vi "Edit.vi"(8 "error in (no error)":errorcluster, 10 "Edit dialog":T1, 11 "Action in":refnum<class "Substrate.lvclass">) -> (0 "error out":errorcluster, 3 "Action out":refnum<class "Substrate.lvclass">)   [LabVIEW 2013, in "PowderDeposition.lvlib" / "Substrate.lvclass"]
uses:
  Substrate.lvclass
  Move-Absolute/Move-Absolute-settings.ctl
  Substrate.lvclass/Substrate.ctl
  Move-Absolute/Move-Absolute.lvclass
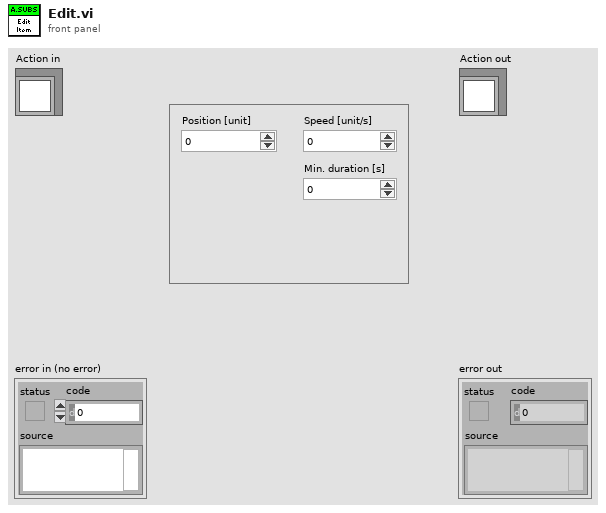
[diagram p1: front panel]
types:
  T1 = typedef "PowderDeposition.lvlib/Move-Absolute.lvclass/Move-Absolute-settings.ctl" = cluster{"Position":dbl, "Speed":dbl, "Min duration":dbl}
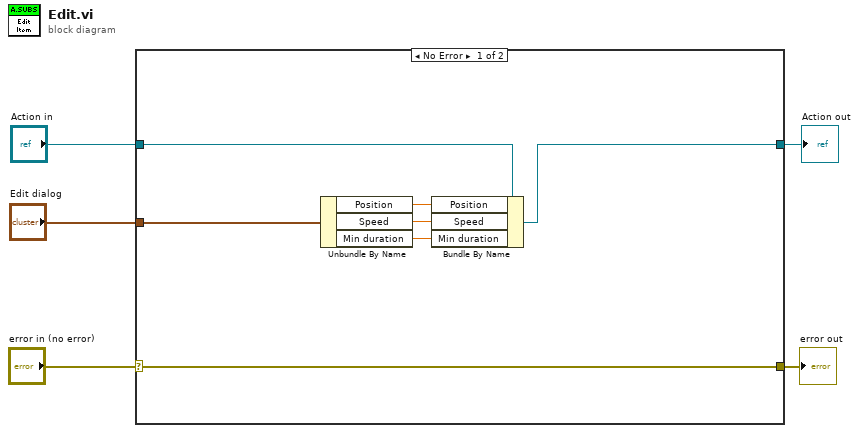
[diagram p0: block diagram]
diagram:
  n1 = case shown="No Error" "error in (no error)" {
    selector: "error in (no error)" -> [w6 w14]
    tunnel: [w6 w14] -> w4
    tunnel: [w7 w13] -> w2
    tunnel: "Action in" -> [w8 w13]
    tunnel: "Edit dialog" -> [w9 _]
    frame No Error {
      n2 = Unbundle By Name(w9) -> ("Position"=w12:dbl, "Speed"=w11:dbl, "Min duration"=w10:dbl)
      n3 = Bundle By Name(cluster=w8, "Position"=w12, "Speed"=w11, "Min duration"=w10) -> (w7:refnum<class "Substrate.lvclass">)
    }
    frame Error {
    }
  }
  "error out" <- w4
  "Action out" <- w2
